vi "ex8-3.vi"   [LabVIEW 2009]
uses:
  <vilib>/NXT/Block Support/NXT_InputPort.ctl
  <vilib>/NXT/Dual Mode Library/Display/drawText.vi
  <vilib>/NXT/Dual Mode Library/Display/drawNumber.vi
  <vilib>/NXT/Dual Mode Library/Sensors/Sonar_cm.vi
types:
  T1 = typedef "NXT_InputPort.ctl" = u8
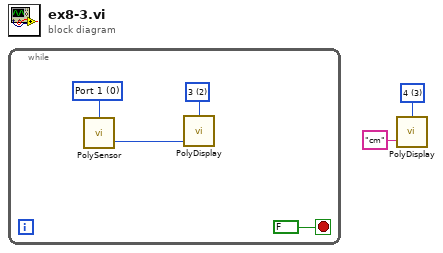
[diagram p0: block diagram]
diagram:
  w2 = i16 3 items=["1", "2", "3", "4", "5", "6", "7", "8"] ("Line")
  n1 = while {
    stop <- FALSE stop-if-true
    w4 = i16 2 items=["1", "2", "3", "4", "5", "6", "7", "8"] ("Line")
    w5 = T1 0 items=["Port 1", "Port 2", "Port 3", "Port 4"] ("Port (Port 4)")
    n2 = call-poly <vilib>:"PolySensor.vi"("Port (Port 4)"=w5) -> ("Distance (cm)"=w3:i16)  [unwired: 2 in, 1 out]
    n3 = call-poly <vilib>:"PolyDisplay.vi"("number"=w3, "Line"=w4) -> ()  [unwired: 2 in, 1 out]
  }
  n4 = call-poly <vilib>:"PolyDisplay.vi"("Text"="cm", "Line"=w2) -> ()  [unwired: 2 in, 1 out]
